vi "myRIO_BRig_RT__Case_Exp_State_ENL1__v3.vi"(7 "I_lick":bool, 8 "input_arrTrig":bool[](array[boolean]), 10 "input_state":T1, 11 "input_dataCurrent":u16[](array[numeric])) -> (0 "output_l1_laserOn":bool, 1 "output_l1_laserEvent":bool, 2 "output_state":T1, 3 "output_dataCurrent":u16[](array[numeric]), 4 "output_l2_laserEvent":bool, 6 "output_l2_laserOn":bool)   [LabVIEW 2014]
uses:
  myRIO_BRig_RT__Case_Exp_stateList.ctl
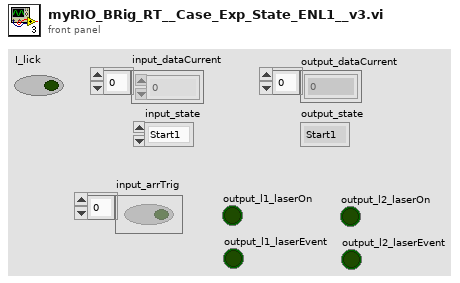
[diagram p1: front panel]
types:
  T1 = typedef "myRIO_BRig_RT__Case_Exp_stateList.ctl" = enum16{"Start1", "Start2", "Start3", "saveSettings1", "saveSettings2", "saveSettings3", "saveSettings4", "saveSettings_LC_ENL_l1", "saveSettings_LC_ENL_l2", "saveSettings_LC_Cue_l1", "saveSettings_LC_Cue_l2", "saveSettings6_LC_l1_Other", "SaveSettings6_LC_l2_Other", "setSettings_Audio", "setSettings_Laser", "initBlock_pre", "initBlock", "initBlock2", "initBlock_post", "initTrial_pre", "initTrial", "initTrial2", "initTrial3", "initTrial4", "initTrial_LC_ENL1", "initTrial_LC_Cue1", "initTrial_LC_Cue1_2", "initTrial_LC_Sel", "initTrial_post", "ENL1_pre", "ENL1", "ENL1_post", "ENL1Penalty_pre", "ENL1Penalty", "ENL2_pre", "ENL2", "ENL2Penalty_pre", "ENL2Penalty", "Cue1_pre", "Cue1", "Cue1_post", "Cue1Penalty_pre", "Cue1Penalty", "Cue2_pre", "Cue2", "Cue2Penalty_pre", "Cue2Penalty", "Selection_pre", "Selection", "Select_post", "SelectReward_pre", "SelectReward", "SelectRewardPost_pre", "SelectRewardPost", "SelectWrong_pre", "SelectWrong", "SelectWrong_post", "SelectTimeout_pre", "SelectTimeout", "SelectTimeout_post", "endTrial_pre", "endTrial1", "endTrial2", "endTrial3", "endTrial_post", "endBlock_pre", "endBlock", "endBlock_post", "endExp", "commConnect", "commUpload_pre", "commUpload_dataBlock", "commUpload_dataCurrent", "commUpload_dataExp", "commUpload_dataLC", "commUpload_dataTrial", "commUpload_post", "saveData_pre", "saveData_dataBlock", "saveData_dataCurrent", "saveData_dataExp", "saveData_dataLC", "saveData_dataTrial", "saveData_post", "empty_endBlock1", "empty_endBlock2", "empty_endTrial1", "empty_endTrial2", "empty_endTrial3", "empty_endTrial4", "empty_endTrial5", "dummyState", "dummyState_endBlock"}
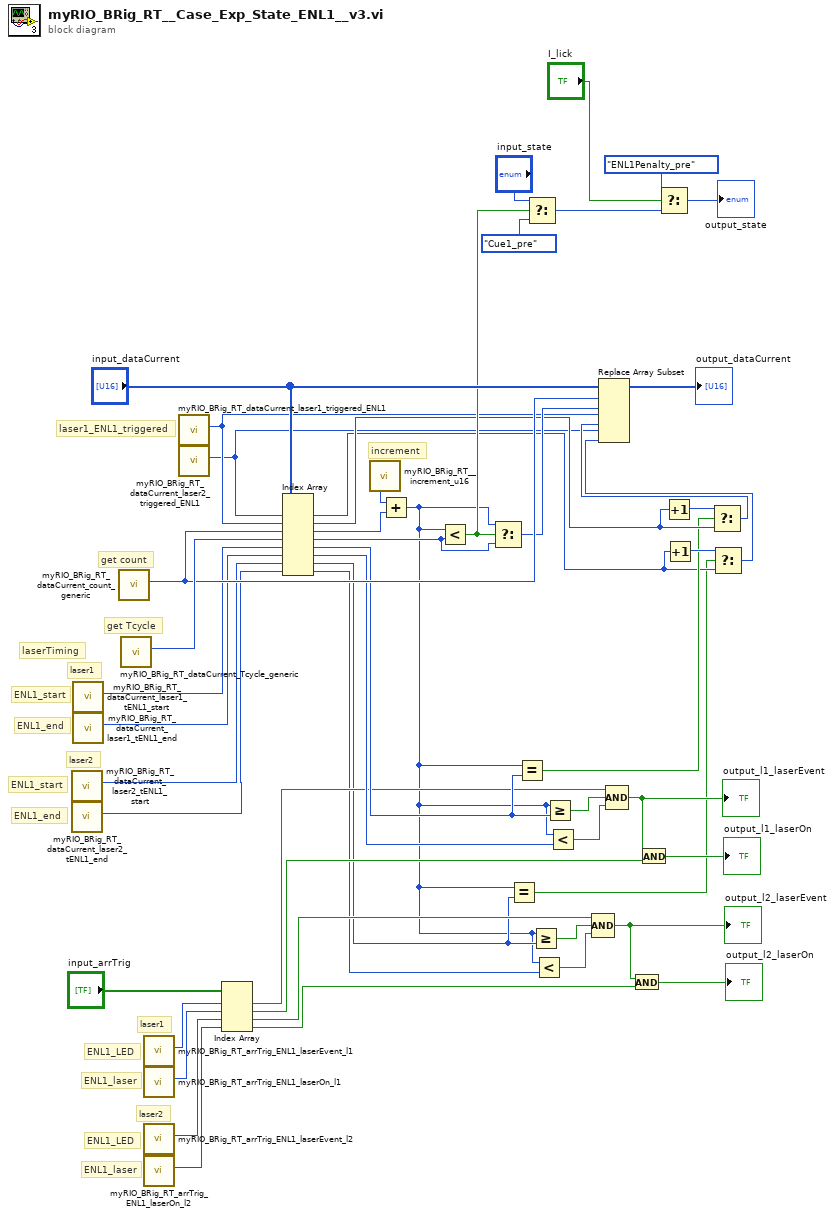
[diagram p0: block diagram]
diagram:
  # "ENL1_LED"
  # "ENL1_laser"
  # "ENL1_LED"
  # "ENL1_laser"
  # "laser2"
  # "laser1"
  # "ENL1_end"
  # "ENL1_start"
  # "laser2"
  # "laser1"
  # "ENL1_end"
  # "ENL1_start"
  # "laser1_ENL1_triggered"
  # "laserTiming"
  # "increment"
  # "get Tcycle"
  # "get count"
  n1 = call "myRIO_BRig_RT_dataCurrent_laser2_tENL1_start.vi"() -> ("output_laser2_tENL1_start"=w10:i32)  [unwired: 11 in]
  n2 = call "myRIO_BRig_RT_dataCurrent_laser2_tENL1_end.vi"() -> ("output_laser2_tENL1_end"=w9:i32)  [unwired: 11 in]
  n3 = call "myRIO_BRig_RT_dataCurrent_laser1_tENL1_start.vi"() -> ("output_laser1_tENL1_start"=w12:i32)  [unwired: 11 in]
  n4 = call "myRIO_BRig_RT_dataCurrent_laser1_tENL1_end.vi"() -> ("output_laser1_tENL1_end"=w11:i32)  [unwired: 11 in]
  n5 = call "myRIO_BRig_RT_dataCurrent_count_generic.vi"() -> ("output_count_generic"=w48:i32)  [unwired: 11 in]
  n6 = call "myRIO_BRig_RT_dataCurrent_Tcycle_generic.vi"() -> ("output_Tcycle_generic"=w49:i32)  [unwired: 11 in]
  n7 = call "myRIO_BRig_RT_arrTrig_ENL1_laserEvent_l1.vi"() -> ("output_arrTrig_ENL1_laserEvent_l1"=w15:i32)  [unwired: 11 in]
  n8 = call "myRIO_BRig_RT_arrTrig_ENL1_laserOn_l1.vi"() -> ("output_arrTrig_ENL1_laserOn_l1"=w16:i32)  [unwired: 11 in]
  n9 = call "myRIO_BRig_RT_arrTrig_ENL1_laserEvent_l2.vi"() -> ("output_arrTrig_ENL1_laserEvent_l2"=w14:i32)  [unwired: 11 in]
  n10 = call "myRIO_BRig_RT_arrTrig_ENL1_laserOn_l2.vi"() -> ("output_arrTrig_ENL1_laserOn_l2"=w13:i32)  [unwired: 11 in]
  n11 = call "myRIO_BRig_RT_dataCurrent_laser1_triggered_ENL1.vi"() -> ("output_laser1_triggered_ENL1"=w17:i32)  [unwired: 11 in]
  n12 = call "myRIO_BRig_RT_dataCurrent_laser2_triggered_ENL1.vi"() -> ("output_laser2_triggered_ENL1"=w6:i32)  [unwired: 11 in]
  n13 = Index Array(array="input_arrTrig", index #1=w15, index #2=w16, index #3=w14, index #4=w13) -> (element #1=w25:bool, element #2=w26:bool, element #3=w24:bool, element #4=w23:bool)
  n14 = Index Array(array="input_dataCurrent", index #1=w6, index #2=w17, index #3=w48, index #4=w49, index #5=w12, index #6=w11, index #7=w10, index #8=w9) -> (element #1=w5:u16, element #2=w31:u16, element #3=w29:u16, element #4=w47:u16, element #5=w28:u16, element #6=w34:u16, element #7=w3:u16, element #8=w22:u16)
  n15 = call "myRIO_BRig_RT__increment_u16.vi"() -> ("output_increment__u16"=w42:u16)  [unwired: 11 in]
  n16 = Add(x=w42, y=w29) -> (x+y=w2:u16)
  n17 = Less?(x=w2, y=w47) -> (x < y?=w44:bool)
  n18 = Select(t=w2, s=w44, f=w47) -> (s? t:f=w46:u16)
  n19 = Equal?(x=w2, y=w3) -> (x = y?=w1:bool)
  n20 = Equal?(x=w2, y=w28) -> (x = y?=w7:bool)
  n21 = Select(t="input_state", s=w44, f=myRIO_BRig_RT__Case_Exp_stateList."Cue1_pre" ("Enum")) -> (s? t:f=w43:T1)
  n22 = Greater Or Equal?(x=w2, y=w3) -> (x >= y?=w21:bool)
  n23 = Less?(x=w2, y=w22) -> (x < y?=w20:bool)
  n24 = Greater Or Equal?(x=w2, y=w28) -> (x >= y?=w40:bool)
  n25 = Less?(x=w2, y=w34) -> (x < y?=w41:bool)
  n26 = Compound Arithmetic op=AND(w24, w21, w20) -> (w19:bool)
  "output_l2_laserEvent" <- w19
  n27 = Compound Arithmetic op=AND(w25, w40, w41) -> (w30:bool)
  "output_l1_laserEvent" <- w30
  n28 = And(x=w19, y=w23) -> (x .and. y?=→"output_l2_laserOn":bool)
  n29 = And(x=w30, y=w26) -> (x .and. y?=→"output_l1_laserOn":bool)
  n30 = Select(t=myRIO_BRig_RT__Case_Exp_stateList."ENL1Penalty_pre" ("Enum"), s="I_lick", f=w43) -> (s? t:f=→"output_state":T1)
  n31 = Increment(x=w31) -> (x+1=w32:u16)
  n32 = Increment(x=w5) -> (x+1=w8:u16)
  n33 = Select(t=w32, s=w7, f=w31) -> (s? t:f=w33:u16)
  n34 = Select(t=w8, s=w1, f=w5) -> (s? t:f=w4:u16)
  n35 = Replace Array Subset(array="input_dataCurrent", new element #1=w46, index #1=w48, new element #2=w33, index #2=w17, new element #3=w4, index #3=w6) -> (→"output_dataCurrent":u16[])
